vi "H5Aget_name.vi"(6 "error in (no error)":errorcluster, 9 "HDF5 Attr Ref":T1) -> (0 "error out":errorcluster, 2 "Name":string, 3 "HDF5 Attr Ref out":T1)   [LabVIEW 2017]
doc: "Gets an attribute name."
uses:
  <vilib>/UPVI/lvhdf5/library.llb/HDF5 Ref.ctl
  <vilib>/UPVI/lvhdf5/hdf5.dll
panel:
  # "LVHDF5 Toolkit\nCopyright (c) 2005-2013 by Jason D. Sommerville\nCopyright (c) 2014 by UPVI, LLC.\n\nThis use and distribution of this file is governed by the terms found in \nLICENSE.txt distributed with this toolkit and installed at\n <user.lib>\\_lvhdf5\\LICENSE.txt"
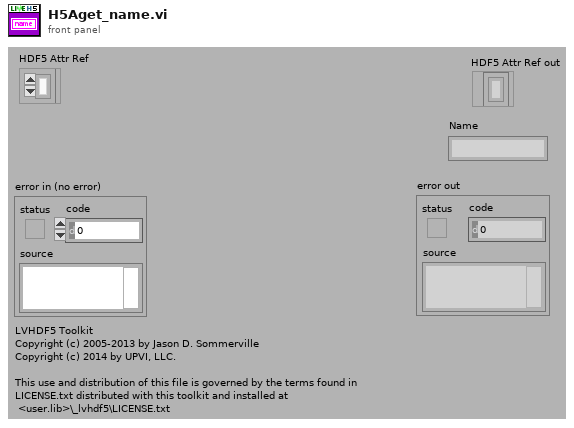
[diagram p1: front panel]
types:
  T1 = typedef "HDF5 Ref.ctl" = refnum<k1>
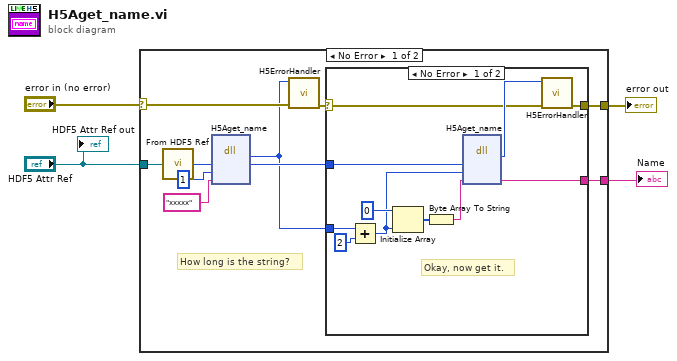
[diagram p0: block diagram]
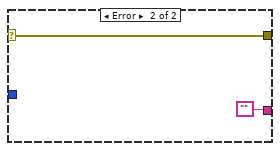
[diagram p2: hidden frame]
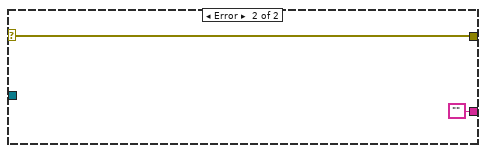
[diagram p3: hidden frame]
diagram:
  n1 = case shown="No Error" "error in (no error)" {
    selector: "error in (no error)" -> [w10 w29]
    tunnel: [w6 w29] -> w2
    tunnel: "HDF5 Attr Ref" -> [w14 _]
    tunnel: [w7 ""] -> w1
    frame No Error {
      # "How long is the string?"
      n2 = call <vilib>:"From HDF5 Ref.vi"("HDF5 Ref"=w14) -> ("I32"=w13:i32)
      n3 = dll-call lib="C:/Program Files/National Instruments/LabVIEW 2017/vi.lib/UPVI/lvhdf5/hdf5.dll" fn="H5Aget_name"("attr_id"=w13, "buf_size"=u32 1, "buf"="xxxxx") -> ("return type"=w5:i64, "attr_id"=w8:i32)  [unwired: 5 in, 2 out]
      n4 = call <vilib>:"H5ErrorHandler.vi"("error in (no error)"=w10, "herr_t"=w5) -> ("error out"=w9:errorcluster)  [unwired: 3 in, 4 out]
      n5 = case shown="No Error" w9 {
        selector: w9 -> [w20 w26]
        tunnel: w5 -> [w17 _]
        tunnel: w8 -> [w22 _]
        tunnel: [w19 w26] -> w6
        tunnel: [w18 ""] -> w7
        frame No Error {
          # "Okay, now get it."
          n6 = Add(x=w17, y=2) -> (x+y=w15:i64)
          n7 = Initialize Array(u8 0, w15) -> (w24:u8[])
          n8 = Byte Array To String(unsigned byte array=w24) -> (string=w23:string)
          n9 = dll-call lib="C:/Program Files/National Instruments/LabVIEW 2017/vi.lib/UPVI/lvhdf5/hdf5.dll" fn="H5Aget_name"("attr_id"=w22, "buf_size"=w15, "buf"=w23) -> ("return type"=w21:i64, "buf"=w18:string)  [unwired: 5 in, 2 out]
          n10 = call <vilib>:"H5ErrorHandler.vi"("error in (no error)"=w20, "herr_t"=w21) -> ("error out"=w19:errorcluster)  [unwired: 3 in, 4 out]
        }
        frame Error {
        }
      }
    }
    frame Error {
    }
  }
  "error out" <- w2
  "Name" <- w1
  "HDF5 Attr Ref out" <- "HDF5 Attr Ref"
